vi "Main.vi"(11 "Module Admin":refnum<class "Delacor_lib_QMH_Module Admin.lvclass">) -> ()   [LabVIEW 2020, in "acquisition.lvlib"]
doc: "This template is based off of the Queued Message Handler design pattern and the Queued Message Handler project template that ships with LabVIEW.\n\nThe main difference is that the queue is private to this module and communication between modules is performed via Broadcast and Request events.\n\nRequest events are wrapped in public API methods and are handled in the Event Handling Loop (EHL) of this VI. Any module can register for Broadcast events sent by this module. The EHL generates messages based on user interface actions.\n\nThe Message Handling Loop (MHL) processes messages generated by the EHL, or by other messages. The messages are string values, so new messages can be added easily to the Message Cases case structure in the MHL. Each message cluster can also provide an optional value for Message Data, which is a variant that can be converted to whatever message-specific data is required.\n_____\nBased on Delacor QMH Project Template 6.0.0.89."
uses:
  Acquisition.lvlib
  <vilib>/Delacor/Delacor QMH/Libraries/Module Admin_class/Delacor_lib_QMH_Module Admin.lvclass
  Module Data--cluster.ctl
  Stop Argument--cluster.ctl
  <vilib>/Delacor/Delacor QMH/Libraries/Message Queue_class/Delacor_lib_QMH_Message Queue.lvclass/Delacor_lib_QMH_Message Queue.ctl
  <vilib>/Delacor/Delacor QMH/Libraries/Module Admin_class/Delacor_lib_QMH_Module Admin.lvclass/Delacor_lib_QMH_Module Admin.ctl
  startAQ Argument--cluster.ctl
  stopAQ Argument--cluster.ctl
  <vilib>/Utility/miscctls.llb/LVPointTypeDef.ctl
  <vilib>/Delacor/Delacor QMH/Libraries/Message Queue_class/Delacor_lib_QMH_Enqueue Message (Single).vi
  <vilib>/Delacor/Delacor QMH/Libraries/Module Admin_class/Delacor_lib_QMH_Get External Launch.vi
  <vilib>/Utility/error.llb/Error Cluster From Error Code.vi
  <vilib>/ErrorRing/Error Ring.xnode
  <vilib>/Delacor/Delacor QMH/Libraries/Message Queue_class/Delacor_lib_QMH_Message Queue.lvclass
  <vilib>/measure/NI_MABase.lvlib
  <vilib>/Analysis/NI_AALBase.lvlib
  UI/UI.lvlib
panel:
  in  "SimulatedData":T1
  out "Waveform Graph":waveform(dbl)(graph)
  out "error out":errorcluster
  out "Status":string
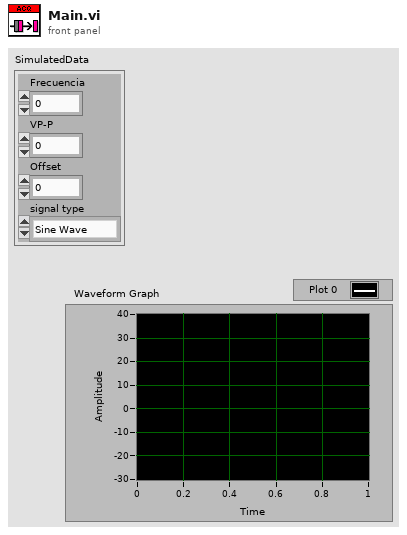
[diagram p1: front panel]
types:
  T1 = cluster{"Frecuencia":dbl, "VP-P":dbl, "Offset":dbl, "signal type":enum16{"Sine Wave", "Triangle Wave", "Square Wave", "Sawtooth Wave"}}
  T2 = typedef "acquisition.lvlib/Request Events--cluster.ctl" = cluster{"Stop Module":refnum<user-event>, "Show Panel":refnum<user-event>, "Hide Panel":refnum<user-event>, "Get Module Execution Status":refnum<user-event>, "Show Diagram":refnum<user-event>, "startAQ":refnum<user-event>, "stopAQ":refnum<user-event>, "StartSimulatedHelperLoop":refnum<user-event>, "StopSimulatedHelperLoop":refnum<user-event>}
  T3 = typedef "UI.lvlib/Broadcast Events--cluster.ctl" = cluster{"Module Did Init":refnum<user-event>, "Status Updated":refnum<user-event>, "Error Reported":refnum<user-event>, "Module Did Stop":refnum<user-event>, "Update Module Execution Status":refnum<user-event>}
  T4 = typedef "acquisition.lvlib/Module Data--cluster.ctl" = cluster{"Status":string, "SimulatedData":cluster{"Frecuencia":dbl, "VP-P":dbl, "Offset":dbl, "signal type":enum16{"Sine Wave", "Triangle Wave", "Square Wave", "Sawtooth Wave"}}}
  T5 = enum32{"invalid lock state", "Not Locked", "Locked (No Password)", "Password-protected"}
  T6 = typedef "acquisition.lvlib/Stop Argument--cluster.ctl" = cluster{"Origin":string, "Exit via Stop Module Req?":bool, "Wait for Module to stop?":bool}
  T7 = typedef "acquisition.lvlib/startAQ Argument--cluster.ctl" = cluster{"Boolean":bool}
  T8 = typedef "acquisition.lvlib/stopAQ Argument--cluster.ctl" = cluster{"Boolean":bool}
  T9 = typedef "LVPointTypeDef.ctl" = cluster{"Horizontal":i16, "Vertical":i16}
  T10 = enum32{"Invalid", "Standard", "Closed", "Hidden", "Minimized", "Maximized"}
  T11 = enum16{"Sine Wave", "Triangle Wave", "Square Wave", "Sawtooth Wave"}
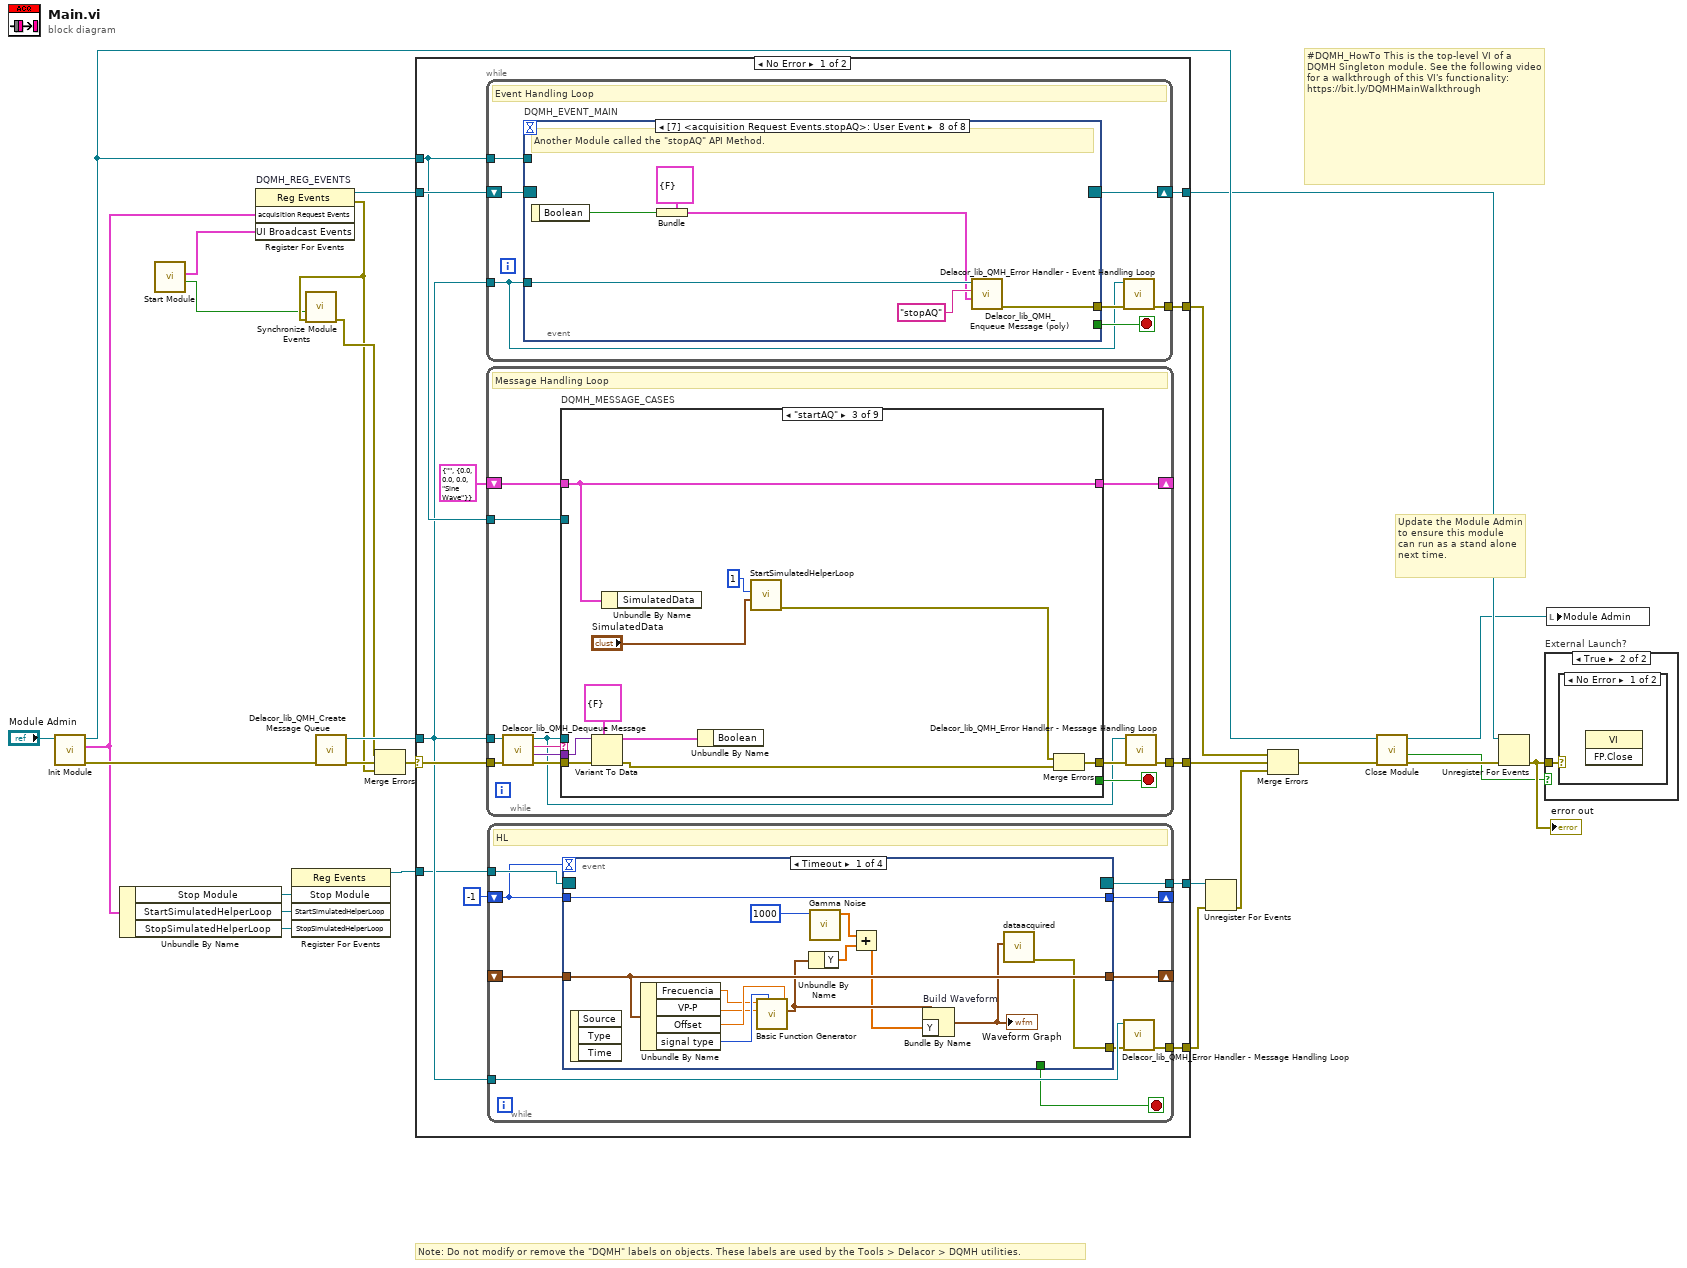
[diagram p0: block diagram]
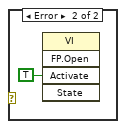
[diagram p3: hidden frame]
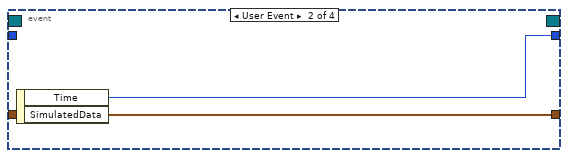
[diagram p4: hidden frame]
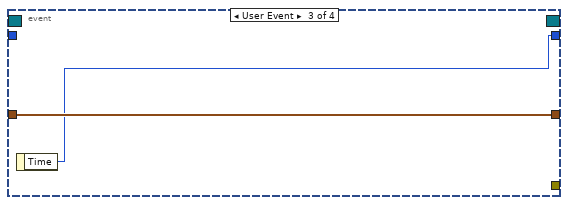
[diagram p5: hidden frame]
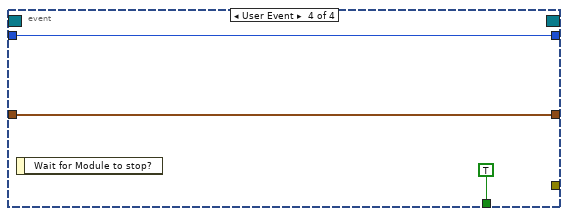
[diagram p6: hidden frame]
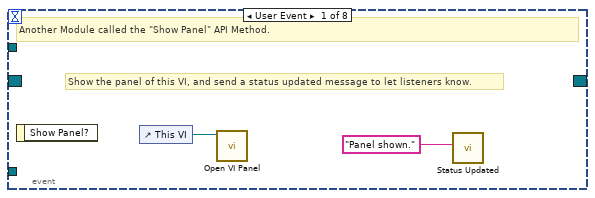
[diagram p7: hidden frame]
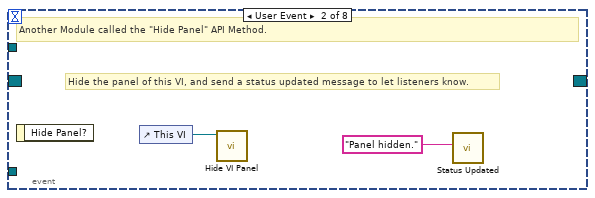
[diagram p8: hidden frame]
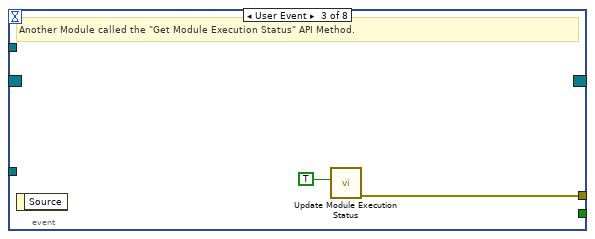
[diagram p9: hidden frame]
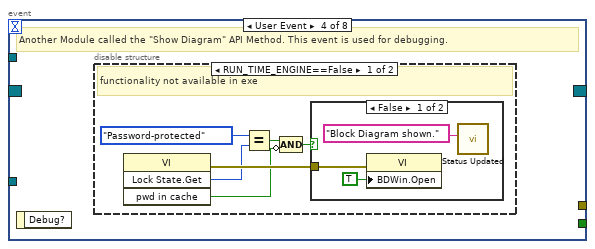
[diagram p10: hidden frame]
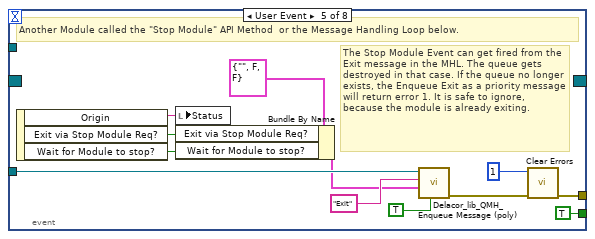
[diagram p13: hidden frame]
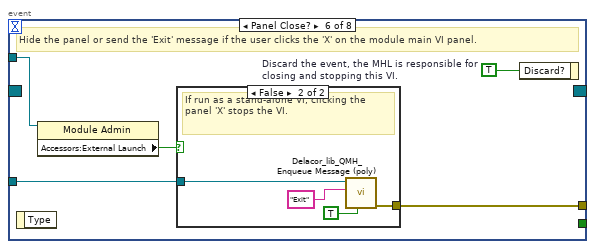
[diagram p14: hidden frame]
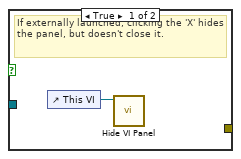
[diagram p15: hidden frame]
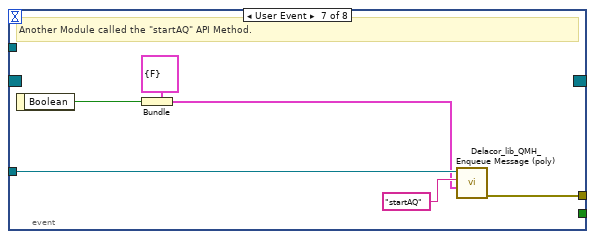
[diagram p16: hidden frame]
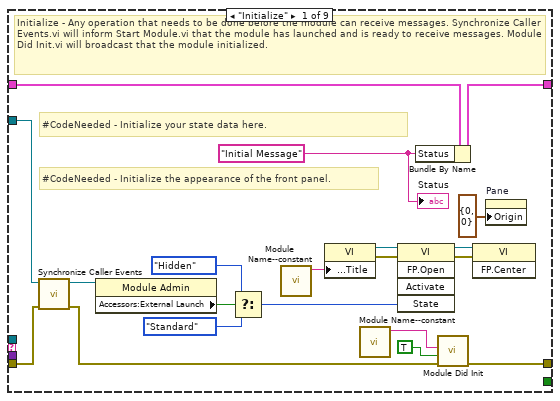
[diagram p17: hidden frame]
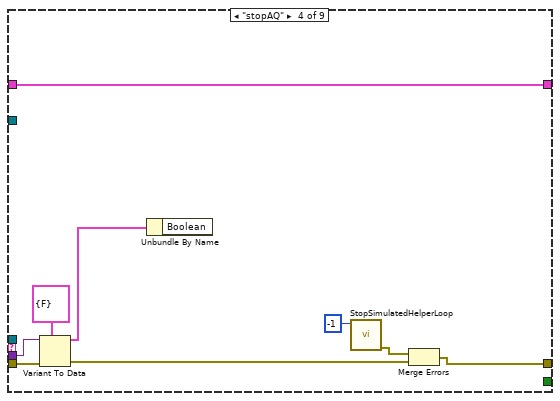
[diagram p19: hidden frame]
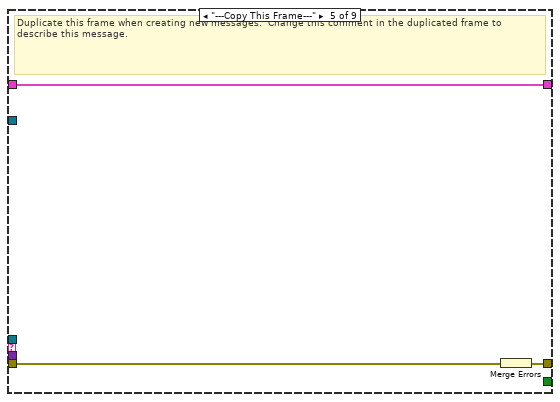
[diagram p20: hidden frame]
diagram:
  # "#DQMH_HowTo This is the top-level VI of a DQMH Singleton module. See the following video for a walkthrough of this VI's functionality: https://bit.ly/DQMHMainWalkthrough"
  # "Note: Do not modify or remove the \"DQMH\" labels on objects. These labels are used by the Tools > Delacor > DQMH utilities."
  # "Update the Module Admin to ensure this module can run as a stand alone next time."
  n1 = call "Init Module.vi"("Singleton Module Admin in"="Module Admin") -> ("error out"=w26:errorcluster, "acquisition Request Events"=w7:T2, "Singleton Module Admin out"=w19:refnum<class "Delacor_lib_QMH_Module Admin.lvclass">)  [unwired: 8 in]
  n2 = Unbundle By Name(w7) -> ("Stop Module"=w8:refnum<user-event>, "StartSimulatedHelperLoop"=w6:refnum<user-event>, "StopSimulatedHelperLoop"=w5:refnum<user-event>)
  n3 = call "Start Module.vi"() -> ("Wait for Event Sync?"=w1:bool, "UI Broadcast Events"=w4:T3)  [unwired: 8 in, 2 out]
  n4 = register-events "DQMH_REG_EVENTS"(w7, w4) -> (reference out=w17:refnum<event-registration>, error out=w2:errorcluster)  [unwired: 2 in]
  n5 = register-events(w8, w6, w5) -> (reference out=w9:refnum<event-registration>)  [unwired: 2 in, 1 out]
  n6 = call "Synchronize Module Events.vi"("error in"=w2, "Wait for Event Sync?"=w1) -> ("error out"=w3:errorcluster)  [unwired: 9 in]
  n7 = call <vilib>:"Delacor_lib_QMH_Create Message Queue.vi"("error in"=w26) -> ("error out"=w21:errorcluster, "Message Queue"=w16:refnum<class "Delacor_lib_QMH_Message Queue.lvclass">)  [unwired: 9 in]
  n8 = Merge Errors(w3, w21, w2) -> (w20:errorcluster)
  n9 = case shown="No Error" w20 {
    selector: w20 -> [w37 w232]
    tunnel: [w39 w231] -> w27
    tunnel: [w36 w237] -> w18
    tunnel: w17 -> [w34 w237]
    tunnel: w16 -> [w31 w230]
    tunnel: [w38 _] -> w24
    tunnel: w19 -> [w33 w233]
    tunnel: [w32 _] -> w11
    tunnel: [w30 w229] -> w10
    tunnel: w9 -> [w29 w229]
    frame No Error {
      n10 = while {
        tunnel: w31 -> [w70]
        shift-right: [w73] -> w36
        shift-left: w34 -> [w74]
        tunnel: [w75] -> w38
        tunnel: w33 -> [w71]
        stop <- w72 stop-if-true
        # "Event Handling Loop"
        n11 = event "DQMH_EVENT_MAIN" shown="[7] <acquisition Request Events.stopAQ>: User Event" {
          selector: w74 -> [_ _ _ _ _ _ _ _]
          dyn-events: [_ _ _ _ _ _ _ _] -> w73
          timeout: _ -> [_ _ _ _ _ _ _ _]
          tunnel: [_ _ _ _ TRUE ("Discard?") _ _ _] -> w72
          tunnel: w70 -> [_ _ _ _ w99 w106 w119 w125]
          tunnel: [_ _ w82 _ w102 w108 w114 w120] -> w76
          tunnel: w71 -> [_ _ _ _ _ w105 _ _]
          event User Event {
            # "Show the panel of this VI, and send a status updated message to let listeners know."
            # "Another Module called the \"Show Panel\" API Method."
            n12 = event-data() -> ()  [unwired: 1 in, 1 out]
            n13 = control-ref of="This VI"() -> (w78:refnum<vi>)
            n14 = call "Open VI Panel.vi"("VI"=w78) -> ()  [unwired: 10 in, 1 out]
            n15 = call "Status Updated.vi"("Status"="Panel shown." ("format string")) -> ()  [unwired: 10 in, 1 out]
          }
          event User Event {
            # "Hide the panel of this VI, and send a status updated message to let listeners know."
            # "Another Module called the \"Hide Panel\" API Method."
            n16 = event-data() -> ()  [unwired: 1 in, 1 out]
            n17 = control-ref of="This VI"() -> (w80:refnum<vi>)
            n18 = call "Hide VI Panel.vi"("VI"=w80) -> ()  [unwired: 10 in, 1 out]
            n19 = call "Status Updated.vi"("Status"="Panel hidden." ("format string")) -> ()  [unwired: 10 in, 1 out]
          }
          event User Event {
            # "Another Module called the \"Get Module Execution Status\" API Method."
            n20 = event-data() -> ()  [unwired: 1 in, 1 out]
            n21 = call "Update Module Execution Status.vi"("Running?"=TRUE) -> ("error out"=w82:errorcluster)  [unwired: 10 in]
          }
          event User Event {
            # "Another Module called the \"Show Diagram\" API Method. This event is used for debugging."
            n22 = event-data() -> ()  [unwired: 1 in, 1 out]
            n23 = disable-structure shown="RUN_TIME_ENGINE==False" {
              frame condition #0 (active) {
                # "functionality not available in exe"
                n24 = invoke class="VI" method="Lock State.Get"() -> (error out=w88:errorcluster, "Get Lock State"=w87:T5, "pwd in cache"=w84:bool)  [unwired: 4 in, 1 out]
                n25 = Equal?(x=T5."Password-protected", y=w87) -> (x = y?=w85:bool)
                n26 = Compound Arithmetic op=AND(w85, invert w84) -> (w83:bool)
                n27 = case shown="False" w83 {
                  tunnel: w88 -> [w91 _]
                  frame False {
                    n28 = property class="VI"(error in=w91, "BDWin.Open"=TRUE ("Block Diagram Window:Open")) -> ()  [unwired: 1 in, 2 out]
                    n29 = call "Status Updated.vi"("Status"="Block Diagram shown." ("format string")) -> ()  [unwired: 10 in, 1 out]
                  }
                  frame True {
                    # "Password-protected VI, and the password is not in the cache. Do not show the diagram."
                  }
                }
              }
              frame condition #1 {
              }
            }
          }
          event User Event {
            # "The Stop Module Event can get fired from the Exit message in the MHL. The queue gets destroyed in that case. If the queue no longer exists, the Enqueue Exit as a priority message will return error 1. It is safe to ignore, because the module is already exiting."
            # "Another Module called the \"Stop Module\" API Method  or the Message Handling Loop below."
            n30 = event-data() -> ("Origin"=w98:string, "Exit via Stop Module Req?"=w94:bool, "Wait for Module to stop?"=w93:bool)  [unwired: 1 in]
            n31 = local write "Status"(w98) -> ()
            n32 = Bundle By Name(cluster=T6 {"Origin"="", "Exit via Stop Module Req?"=FALSE, "Wait for Module to stop?"=FALSE} ("Stop Argument"), "Exit via Stop Module Req?"=w94, "Wait for Module to stop?"=w93) -> (w92:T6)
            n33 = call-poly <vilib>:"Delacor_lib_QMH_Enqueue Message (poly).vi"("Priority Message? (F)"=TRUE, "Message Data"=w92, "Message"="Exit", "Message Queue in"=w99) -> ("error out"=w103:errorcluster)  [unwired: 6 in, 1 out]
            n34 = call <vilib>:"Clear Errors.vi"("error in (no error)"=w103, "specific error code to clear (0: all)"=1) -> ("error out"=w102:errorcluster)  [unwired: 4 in, 1 out]
          }
          event Panel Close? {
            w107 = TRUE  # Discard the event, the MHL is responsible for closing and stopping this VI.
            # "Hide the panel or send the 'Exit' message if the user clicks the 'X' on the module main VI panel."
            n35 = event-data() -> ()  [unwired: 1 in, 1 out]
            n36 = property class="Module Admin"(reference=w105) -> ("Accessors:External Launch"=w104:bool)  [unwired: 1 in, 2 out]
            n37 = case shown="False" w104 {
              tunnel: w106 -> [_ w112]
              tunnel: [_ w113] -> w108
              frame True {
                # "If externally launched, clicking the 'X' hides the panel, but doesn't close it."
                n38 = control-ref of="This VI"() -> (w109:refnum<vi>)
                n39 = call "Hide VI Panel.vi"("VI"=w109) -> ()  [unwired: 10 in, 1 out]
              }
              frame False {
                # "If run as a stand-alone VI, clicking the panel 'X' stops the VI."
                n40 = call-poly <vilib>:"Delacor_lib_QMH_Enqueue Message (poly).vi"("Priority Message? (F)"=TRUE, "Message"="Exit", "Message Queue in"=w112) -> ("error out"=w113:errorcluster)  [unwired: 7 in, 1 out]
              }
            }
            n41 = event-data("Discard?"=w107) -> ()  [unwired: 1 in, 1 out]
          }
          event User Event {
            # "Another Module called the \"startAQ\" API Method."
            n42 = event-data() -> ("Boolean"=w115:bool)  [unwired: 1 in]
            n43 = Bundle(cluster=T7 {"Boolean"=FALSE} ("startAQ Argument"), "Boolean"=w115) -> (w116:T7)
            n44 = call-poly <vilib>:"Delacor_lib_QMH_Enqueue Message (poly).vi"("Message Data"=w116, "Message"="startAQ", "Message Queue in"=w119) -> ("error out"=w114:errorcluster)  [unwired: 7 in, 1 out]
          }
          event User Event {
            # "Another Module called the \"stopAQ\" API Method."
            n45 = event-data() -> ("Boolean"=w121:bool)  [unwired: 1 in]
            n46 = Bundle(cluster=T8 {"Boolean"=FALSE} ("stopAQ Argument"), "Boolean"=w121) -> (w122:T8)
            n47 = call-poly <vilib>:"Delacor_lib_QMH_Enqueue Message (poly).vi"("Message Data"=w122, "Message"="stopAQ", "Message Queue in"=w125) -> ("error out"=w120:errorcluster)  [unwired: 7 in, 1 out]
          }
        }
        n48 = call-dynamic "Delacor_lib_QMH_Error Handler - Event Handling Loop.vi"("error in"=w76, "Message Queue in"=w70) -> ("dup error in"=w75:errorcluster)  [unwired: 8 in, 1 out]
      }
      n49 = while {
        tunnel: w31 -> [w128]
        shift-right: [w132] -> _
        shift-left: T4 {"Status"="", "SimulatedData"={"Frecuencia"=0.0, "VP-P"=0.0, "Offset"=0.0, "signal type"=enum."Sine Wave"}} ("Data Cluster") -> [w133]
        tunnel: w37 -> [w136]
        tunnel: [w134] -> w39
        tunnel: w33 -> [w127]
        stop <- w131 stop-if-true
        # "Message Handling Loop"
        n50 = call-dynamic "Delacor_lib_QMH_Dequeue Message.vi"("error in"=w136, "Message Queue in"=w128) -> ("error out"=w135:errorcluster, "Message Data"=w129:variant, "Message"=w130:string, "Message Queue out"=w126:refnum<class "Delacor_lib_QMH_Message Queue.lvclass">)  [unwired: 6 in]
        n51 = case "DQMH_MESSAGE_CASES" shown="\"startAQ\"" w130 {
          selector: w130 -> [_ _ _ _ _ _ _ _ w216]
          tunnel: w126 -> [_ _ _ _ _ _ w186 w208 _]
          tunnel: w135 -> [w155 w159 w169 w178 w181 w183 w193 w214 w218]
          tunnel: [w153 w159 w164 w172 w180 w183 w189 w211 w219] -> w137
          tunnel: w133 -> [w144 w158 w165 w177 w179 w182 w188 w207 w217]
          tunnel: [w143 w158 w165 w177 w179 w182 w188 w207 w217] -> w132
          tunnel: [_ _ _ _ _ _ _ w206 _] -> w131
          tunnel: w129 -> [_ _ w168 w176 _ _ w187 w205 _]
          tunnel: w127 -> [w145 _ _ _ _ _ w185 w200 _]
          frame "Initialize" {
            w139 = "Initial Message" ("Initial Message")
            # "#CodeNeeded - Initialize the appearance of the front panel."
            # "#CodeNeeded - Initialize your state data here."
            # "Initialize - Any operation that needs to be done before the module can receive messages. Synchronize Caller Events.vi will inform Start Module.vi that the module has launched and is ready to receive messages. Module Did Init.vi will broadcast that the module initialized."
            n52 = call "Synchronize Caller Events.vi"("error in (no error)"=w155, "Singleton Module Admin in"=w145) -> ("error out"=w154:errorcluster, "Singleton Module Admin out"=w140:refnum<class "Delacor_lib_QMH_Module Admin.lvclass">)  [unwired: 8 in]
            n53 = property class="Module Admin"(reference=w140) -> ("Accessors:External Launch"=w149:bool)  [unwired: 1 in, 2 out]
            n54 = Select(t=T10."Hidden" ("State"), s=w149, f=T10."Standard" ("State")) -> (s? t:f=w146:T10)
            n55 = call "Module Name--constant.vi"() -> ("Module Name"=w152:string)  [unwired: 11 in]
            n56 = property class="VI"("Front Panel.Title"=w152) -> (reference out=w151:refnum<vi>, error out=w157:errorcluster)  [unwired: 2 in]
            n57 = call "Module Name--constant.vi"() -> ("Module Name"=w141:string)  [unwired: 11 in]
            n58 = invoke class="VI" method="FP.Open"(reference=w151, error in=w157, "State"=w146) -> (reference out=w150:refnum<vi>, error out=w156:errorcluster)  [unwired: 2 in, 3 out]
            n59 = Bundle By Name(cluster=w144, "Status"=w139) -> (w143:T4)
            n60 = call "Module Did Init.vi"("error in (no error)"=w154, "Initialized?"=TRUE, "Origin"=w141) -> ("error out"=w153:errorcluster)  [unwired: 8 in]
            n61 = invoke class="VI" method="FP.Center"(reference=w150, error in=w156) -> ()  [unwired: 1 in, 3 out]
            n62 = property on="Pane" class="Pane"("Origin"=T9 {"Horizontal"=0, "Vertical"=0}) -> ()  [unwired: 2 in, 2 out]
            "Status" <- w139
          }
          frame "---Module Specific---" {
            # "Separator -- The following cases handle messages specific to this Module."
          }
          frame "startAQ" {
            n63 = Variant To Data(error in=w169, type=T7 {"Boolean"=FALSE} ("startAQ Argument"), Variant=w168) -> (data=w166:T7, error out=w163:errorcluster)
            n64 = Unbundle By Name(w165) -> ()  [unwired: 1 out]
            n65 = Unbundle By Name(w166) -> ()  [unwired: 1 out]
            n66 = call "StartSimulatedHelperLoop.vi"("SimulatedData"="SimulatedData", "Time"=1) -> ("error out"=w162:errorcluster)  [unwired: 9 in]
            n67 = Merge Errors(w162, w163) -> (w164:errorcluster)
          }
          frame "stopAQ" {
            n68 = Variant To Data(error in=w178, type=T8 {"Boolean"=FALSE} ("stopAQ Argument"), Variant=w176) -> (data=w174:T8, error out=w171:errorcluster)
            n69 = Unbundle By Name(w174) -> ()  [unwired: 1 out]
            n70 = call "StopSimulatedHelperLoop.vi"("Time"=-1) -> ("error out"=w173:errorcluster)  [unwired: 10 in]
            n71 = Merge Errors(w173, w171) -> (w172:errorcluster)
          }
          frame "---Copy This Frame---" {
            # "Duplicate this frame when creating new messages.  Change this comment in the duplicated frame to describe this message."
            n72 = Merge Errors(w181) -> (w180:errorcluster)
          }
          frame "---Exit and Error Handling---" {
            # "Separator - The following cases handle errors and exit messages."
          }
          frame "Error" {
            # "#CodeRecommended - If you ever change the name of this \"Error\" message, you'll need to update the name in the Check Loop Error.vi as well."
            # "#CodeRecommended - If the module is running in standalone mode (External Launch = FALSE), this code will pop up an error dialog and call the 'Exit' message if an error occurs. Add more fine-grained error handling here."
            # "Error - Check the error message data and respond accordingly. This message is sent by the \"Error Handler\" VIs at the end of each loop in this application."
            n73 = property class="Module Admin"(reference=w185) -> ("Accessors:External Launch"=w184:bool)  [unwired: 1 in, 2 out]
            n74 = Variant To Data(error in=w193, type=errorcluster {"status"=FALSE, "code"=0, "source"=""} ("error constant"), Variant=w187) -> (data=w194:errorcluster, error out=w191:errorcluster)
            n75 = call "Error Reported.vi"("Error"=w194) -> ()  [unwired: 10 in, 1 out]
            n76 = case shown="False" w184 {
              tunnel: [w199 _] -> w190
              tunnel: w186 -> [w197 _]
              tunnel: w194 -> [w198 _]
              frame False {
                # "If the module is running standalone, then pop up an error dialog and call the \"Exit\" message."
                n77 = call <vilib>:"Simple Error Handler.vi"("error in (no error)"=w198) -> ()  [unwired: 4 in, 5 out]
                n78 = call-poly <vilib>:"Delacor_lib_QMH_Enqueue Message (poly).vi"("Priority Message? (F)"=TRUE, "Message"="Exit", "Message Queue in"=w197) -> ("error out"=w199:errorcluster)  [unwired: 7 in, 1 out]
              }
              frame True {
                # "If the module was launched externally, calling the Error Reported broadcast VI is the only action performed by the \"Error\" message. The module's caller can then process the error appropriately."
              }
            }
            n79 = Merge Errors(w191, w190) -> (w189:errorcluster)
            n80 = local write "error out"(w189) -> ()
          }
          frame "Exit" {
            w204 = 91  # 91: not all Exit messages will have an argument
            w206 = TRUE  # Stop the VI
            # "Release the message queue reference"
            # "#CodeNeeded - Add any required cleanup code here"
            # "Exit - Exit the application."
            n81 = Variant To Data(error in=w214, type=T6 {"Origin"="", "Exit via Stop Module Req?"=FALSE, "Wait for Module to stop?"=FALSE} ("Stop Argument"), Variant=w205) -> (data=w202:T6, error out=w210:errorcluster)
            n82 = call <vilib>:"Clear Errors.vi"("error in (no error)"=w210, "specific error code to clear (0: all)"=w204) -> ("error out"=w213:errorcluster)  [unwired: 4 in, 1 out]
            n83 = control-ref of="This VI"() -> (w201:refnum<vi>)
            n84 = call-dynamic "Delacor_lib_QMH_Release Message Queue.vi"("error in"=w213, "Message Queue"=w208) -> ("error out"=w212:errorcluster)  [unwired: 9 in]
            n85 = call "Handle Exit.vi"("Stop Argument"=w202, "Admin in"=w200, "VI reference"=w201) -> ("error out"=w209:errorcluster)  [unwired: 7 in, 1 out]
            n86 = Merge Errors(w212, w209) -> (w211:errorcluster)
          }
          frame Default {
            # "'Default' case only runs if there is a message that isn't defined in any of the other cases.  Output a programming error."
            n87 = call "Module Name--constant.vi"() -> ("Module Name"=w215:string)  [unwired: 11 in]
            n88 = xnode "Error Ring"("parameter 0"=w216, "parameter 1"=w215) -> ("error out"=w220:errorcluster)
            n89 = Merge Errors(w218, w220) -> (w219:errorcluster)
          }
        }
        n90 = call-dynamic "Delacor_lib_QMH_Error Handler - Message Handling Loop.vi"("error in"=w137, "Message Queue in"=w126) -> ("dup error in"=w134:errorcluster)  [unwired: 8 in, 1 out]
      }
      n91 = while {
        tunnel: [w49] -> w32
        tunnel: w31 -> [w48]
        tunnel: [w47] -> w30
        tunnel: w29 -> [w46]
        shift-right: [w43] -> _
        shift-left: -1 -> [w44]
        shift-right: [w42] -> _
        shift-left: _ -> [w41]
        stop <- w45 stop-if-true
        # "HL"
        n92 = event shown="[0] Timeout" {
          selector: w46 -> [_ _ _ _]
          dyn-events: [_ _ _ _] -> w47
          timeout: w44 -> [_ _ _ _]
          tunnel: [_ _ _ TRUE] -> w45
          tunnel: w44 -> [w62 _ _ w68]
          tunnel: [w62 w63 w65 w68] -> w43
          tunnel: [w61 w64 w66 w67] -> w42
          tunnel: w41 -> [w61 _ w66 w67]
          tunnel: [w50 _ _ _] -> w40
          event Timeout {
            n93 = event-data() -> ()  [unwired: 1 in, 3 out]
            n94 = Unbundle By Name(w61) -> ("Frecuencia"=w58:dbl, "VP-P"=w57:dbl, "Offset"=w59:dbl, "signal type"=w60:T11)
            n95 = call <vilib>:"Basic Function Generator.vi"("offset"=w59, "signal type"=w60, "amplitude"=w57, "frequency"=w58) -> ("signal out"=w53:waveform(dbl))  [unwired: 5 in, 2 out]
            n96 = Unbundle By Name ("Get Waveform Components")(w53) -> ("Y"=w54:dbl[])
            n97 = call <vilib>:"Gamma Noise.vi"("samples"=1000) -> ("gamma noise"=w55:dbl[])  [unwired: 9 in, 1 out]
            n98 = Add(x=w55, y=w54) -> (x+y=w52:dbl[])
            n99 = Bundle By Name "Build Waveform"(cluster=w53, "Y"=w52) -> (w51:waveform(dbl))
            "Waveform Graph" <- w51
            n100 = call "dataacquired.vi"("waveform"=w51) -> ("error out"=w50:errorcluster)  [unwired: 10 in]
          }
          event User Event {
            n101 = event-data() -> ("Time"=w63:i32, "SimulatedData"=w64:T1)  [unwired: 1 in]
          }
          event User Event {
            n102 = event-data() -> ("Time"=w65:i32)  [unwired: 1 in]
          }
          event User Event {
            n103 = event-data() -> ()  [unwired: 1 in, 1 out]
          }
        }
        n104 = call-dynamic "Delacor_lib_QMH_Error Handler - Message Handling Loop.vi"("error in"=w40, "Message Queue in"=w48) -> ("dup error in"=w49:errorcluster)  [unwired: 8 in, 1 out]
      }
    }
    frame Error {
      # "Synchronize Caller Events.vi will inform Start Module.vi that the module has launched and will let the code calling Start Module.vi register for broadcasts and would permit the caller receive the broadcast that an error occurred at launch time."
      n105 = call-dynamic "Delacor_lib_QMH_Release Message Queue.vi"("error in"=w232, "Message Queue"=w230) -> ("error out"=w231:errorcluster)  [unwired: 9 in]
      n106 = call "Synchronize Caller Events.vi"("Singleton Module Admin in"=w233) -> ("error out"=w238:errorcluster)  [unwired: 9 in, 1 out]
      n107 = call "Module Name--constant.vi"() -> ("Module Name"=w236:string)  [unwired: 11 in]
      n108 = Format Into String(format string="An error occurred during initialization. %s is no longer running.", w236) -> (resulting string=w234:string)  [unwired: 2 in, 1 out]
      n109 = Merge Errors(w231, w238) -> (w239:errorcluster)
      n110 = call "Error Reported.vi"("Additional Information"=w234, "Error"=w239) -> ()  [unwired: 9 in, 1 out]
    }
  }
  n111 = Unregister For Events(event registration refnum=w10, error in=w11) -> (error out=w12:errorcluster)
  n112 = Merge Errors(w24, w27, w12) -> (w23:errorcluster)
  n113 = call "Close Module.vi"("error in (no error)"=w23, "Module Admin in"=w19) -> ("error out"=w25:errorcluster, "External Launch"=w13:bool, "Module Admin out"=w14:refnum<class "Delacor_lib_QMH_Module Admin.lvclass">)  [unwired: 7 in]
  n114 = Unregister For Events(event registration refnum=w18, error in=w25) -> (error out=w22:errorcluster)
  "error out" <- w22
  n115 = case "External Launch?" shown="True" w13 {
    tunnel: w22 -> [_ w240]
    frame False {
    }
    frame True {
      n116 = case shown="No Error" w240 {
        frame No Error {
          n117 = invoke class="VI" method="FP.Close"() -> ()  [unwired: 3 in, 3 out]
        }
        frame Error {
          n118 = invoke class="VI" method="FP.Open"("Activate"=TRUE ("Activate?")) -> ()  [unwired: 4 in, 5 out]
        }
      }
    }
  }
  n119 = local write "Module Admin"(w14) -> ()
